vi "OAT Convert Speed Waveform to Speed Profile.vi"(0 "speed waveform":waveform(dbl)={"t0"=timestamp(0 s since 1904-01-01), "dt"=0.0, "Y"=[]}, 1 "reset? (F)":bool, 7 "pulse/revolution (1)":i32=1, 11 "error in (no error)":errorcluster) -> (4 "speed profile":T1 {"speed [RPM]" format="%.2f"; "time [s]" format="%.2f"}, 15 "error out":errorcluster)   [LabVIEW 2017, in "SoundVib_TachProcess.lvlib"]
doc: "Use this VI to convert a saved history of speed data sampled at regular time intervals to a speed profile suitable for order analysis with the Sound and Vibration Measurement Suite VIs."
uses:
  <vilib>/addons/Sound and Vibration/Order Analysis/Tach Process/SoundVib_TachProcess.lvlib
  <vilib>/addons/Sound and Vibration/Order Analysis/Tach Process/SubVIs/speed profile.ctl
  <vilib>/addons/_NISVFA/_Shared subVIs/Common/svc_Check for Waveform Parameter Continuity (no state).vi
  <vilib>/addons/_NISVFA/_Shared subVIs/Common/svc_Get SV Channel Info.vi
  <vilib>/addons/_NISVFA/_Shared subVIs/Common/svc_Engineering Units to Unit Label.vi
  <vilib>/addons/_NISVFA/_Shared subVIs/Common/svc_Unit Label to Engineering Units.vi
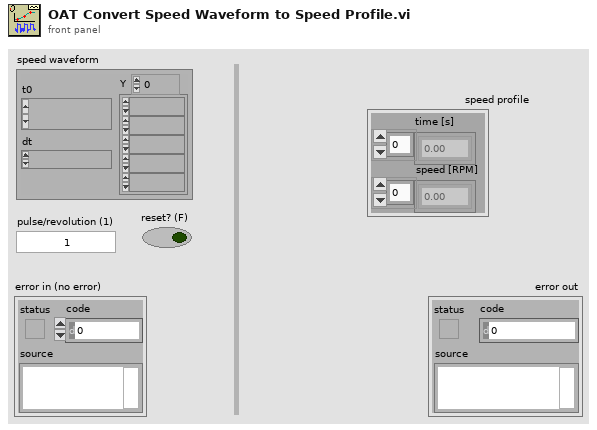
[diagram p1: front panel]
types:
  T1 = typedef "SoundVib_TachProcess.lvlib/speed profile.ctl" = cluster{"time [s]":dbl[], "speed [RPM]":dbl[]}
  T2 = cluster{"dt":bool, "t0 continuity":bool, "array length":bool, "channel info":bool, "name":bool}
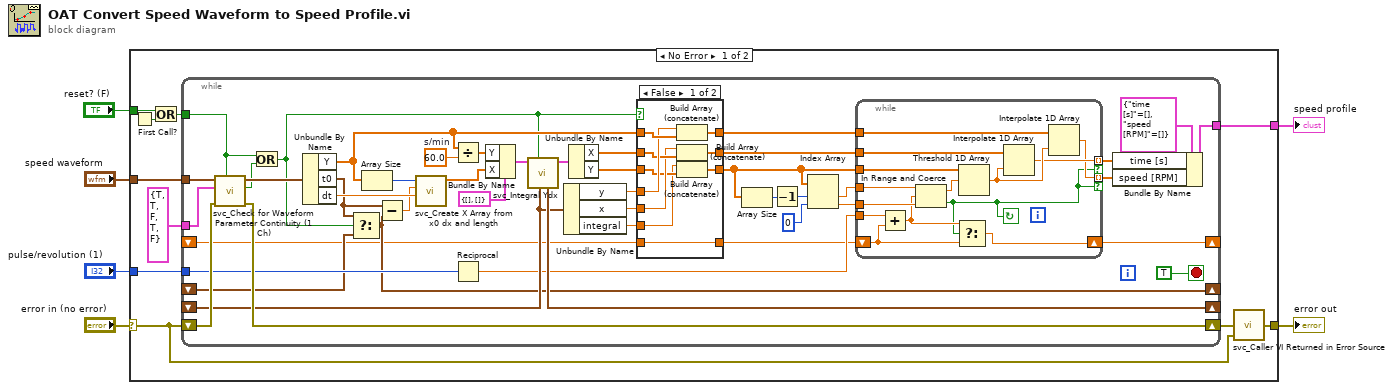
[diagram p0: block diagram]
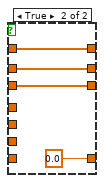
[diagram p2: hidden frame]
diagram:
  n1 = case shown="No Error" "error in (no error)" {
    selector: "error in (no error)" -> [w11 w91]
    tunnel: "speed waveform" -> [w12 _]
    tunnel: [w13 _] -> w5
    tunnel: "pulse/revolution (1)" -> [w16 _]
    tunnel: "reset? (F)" -> [w8 _]
    tunnel: [w14 w91] -> w1
    frame No Error {
      n2 = First Call?() -> (First Call?: T/F=w7:bool)
      n3 = Or(x=w8, y=w7) -> (x .or. y?=w10:bool)
      n4 = while {
        tunnel: w16 -> [w51]
        tunnel: [w36] -> w13
        tunnel: w12 -> [w59]
        shift-right: [w53] -> _
        shift-left: _ -> [w50]
        tunnel: w10 -> [w41]
        tunnel: T2 {"dt"=TRUE, "t0 continuity"=TRUE, "array length"=FALSE, "channel info"=TRUE, "name"=FALSE} ("checks for channel parameter change") -> [w58]
        shift-right: [w38] -> _
        shift-left: _ -> [w39]
        shift-right: [w20] -> _
        shift-left: _ -> [w19]
        shift-right: [w56] -> w15
        shift-left: w11 -> [w57]
        stop <- TRUE stop-if-true
        w43 = 60.0  # s/min
        n5 = call <vilib>:"svc_Check for Waveform Parameter Continuity (1 Ch).vi"("restart averaging (F)"=w41, "error in (no error)"=w57, "checks for channel parameter change"=w58, "scaled signal [EU]"=w59) -> ("error out"=w56:errorcluster, "waveform parameter changed"=w42:bool, "dup scaled signal [EU]"=w45:waveform(dbl))  [unwired: 2 in, 3 out]
        n6 = Or(x=w41, y=w42) -> (x .or. y?=w17:bool)
        n7 = Unbundle By Name(w45) -> ("Y"=w34:dbl[], "t0"=w40:timestamp, "dt"=w60:dbl)
        n8 = Select(t=w40, s=w17, f=w39) -> (s? t:f=w38:timestamp)
        n9 = Array Size(array=w34) -> (size(s)=w62:i32)
        n10 = Subtract(x=w40, y=w38) -> (x-y=w37:dbl)
        n11 = call <vilib>:"svc_Create X Array from x0 dx and length.vi"("dx"=w60, "x0"=w37, "length"=w62) -> ("X"=w27:dbl[])  [unwired: 8 in]
        n12 = Divide(x=w34, y=w43) -> (x/y=w44:dbl[])
        n13 = Reciprocal(x=w51) -> (1/x=w49:dbl)
        n14 = Bundle By Name(cluster=cluster{"X":dbl[], "Y":dbl[]} {"X"=[], "Y"=[]} ("XY"), "Y"=w44, "X"=w27) -> (w54:cluster{"X":dbl[], "Y":dbl[]})
        n15 = call <vilib>:"svc_Integral Ydx.vi"("state in"=w50, "reset"=w17, "XY"=w54) -> ("Integral"=w52:cluster{"X":dbl[], "Y":dbl[]}, "state out"=w53:cluster{"x":dbl, "y":dbl, "integral":dbl})  [unwired: 7 in]
        n16 = Unbundle By Name(w50) -> ("y"=w33:dbl, "x"=w30:dbl, "integral"=w28:dbl)
        n17 = Unbundle By Name(w52) -> ("X"=w31:dbl[], "Y"=w29:dbl[])
        n18 = case shown="False" w17 {
          tunnel: [w84 w90] -> w35
          tunnel: w34 -> [w86 w90]
          tunnel: w33 -> [w85 _]
          tunnel: [w81 w89] -> w32
          tunnel: w31 -> [w83 w89]
          tunnel: w30 -> [w82 _]
          tunnel: [w80 w88] -> w25
          tunnel: w29 -> [w79 w88]
          tunnel: w28 -> [w78 _]
          tunnel: w19 -> [w77 _]
          tunnel: [w77 0.0] -> w18
          frame False {
            n19 = Build Array (concatenate)(w85, w86) -> (w84:dbl[])
            n20 = Build Array (concatenate)(w82, w83) -> (w81:dbl[])
            n21 = Build Array (concatenate)(w78, w79) -> (w80:dbl[])
          }
          frame True {
          }
        }
        n22 = Array Size(array=w25) -> (size(s)=w26:i32)
        n23 = Decrement(x=w26) -> (x-1=w24:i32)
        n24 = Index Array(array=w25, index #1=w24, index #2=0 ("index")) -> (element #1=w22:dbl, element #2=w21:dbl)
        n25 = while {
          tunnel: w25 -> [w76]
          tunnel: w49 -> [w67]
          tunnel: w32 -> [w75]
          tunnel: w35 -> [w74]
          tunnel: [w72] -> w47 mode=indexing if=w63
          tunnel: [w71] -> w46 mode=indexing if=w63
          shift-right: [w64] -> w20
          shift-left: w18 -> [w65]
          tunnel: w22 -> [w70]
          tunnel: w21 -> [w69]
          stop <- w63 continue-if-true
          n26 = Add(x=w67, y=w65) -> (x+y=w66:dbl)
          n27 = In Range and Coerce(upper limit=w70, x=w66, lower limit=w69) -> (coerced(x)=w68:dbl, In Range?=w63:bool)
          n28 = Select(t=w66, s=w63, f=w65) -> (s? t:f=w64:dbl)
          n29 = Threshold 1D Array(2:w68, 3:w76) -> (0:w73:dbl)  [unwired: 1 in]
          n30 = Interpolate 1D Array(1:w73, 2:w75) -> (0:w72:dbl)
          n31 = Interpolate 1D Array(1:w73, 2:w74) -> (0:w71:dbl)
        }
        n32 = Bundle By Name(cluster=T1 {"time [s]"=[], "speed [RPM]"=[]} ("speed profile"), "time [s]"=w47, "speed [RPM]"=w46) -> (w36:T1)
      }
      n33 = call <vilib>:"svc_Caller VI Returned in Error Source.vi"("warning input to caller"=w11, "error in (no error)"=w15) -> ("error out"=w14:errorcluster)  [unwired: 3 in]
    }
    frame Error {
    }
  }
  "error out" <- w1
  "speed profile" <- w5
